vi "2NNN.vi"(11 "Variables and Memory in":T1 {"GFX" format="%02x"}) -> (3 "Variables and Memory out":T1 {"GFX" format="%02x"})   [LabVIEW 2021]
uses:
  Controls/ClusterF.ctl
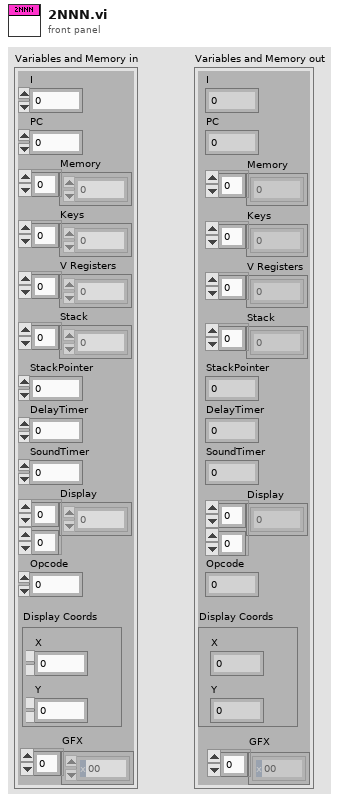
[diagram p1: front panel]
types:
  T1 = typedef "ClusterF.ctl" = cluster{"I":u16, "PC":u16, "Memory":u8[], "Keys":u8[], "V Registers":u8[], "Stack":u16[], "StackPointer":u16, "DelayTimer":u8, "SoundTimer":u8, "Display":u8[][], "Opcode":u16, "Display Coords":cluster{"X":u8, "Y":u8}, "GFX":u8[]}
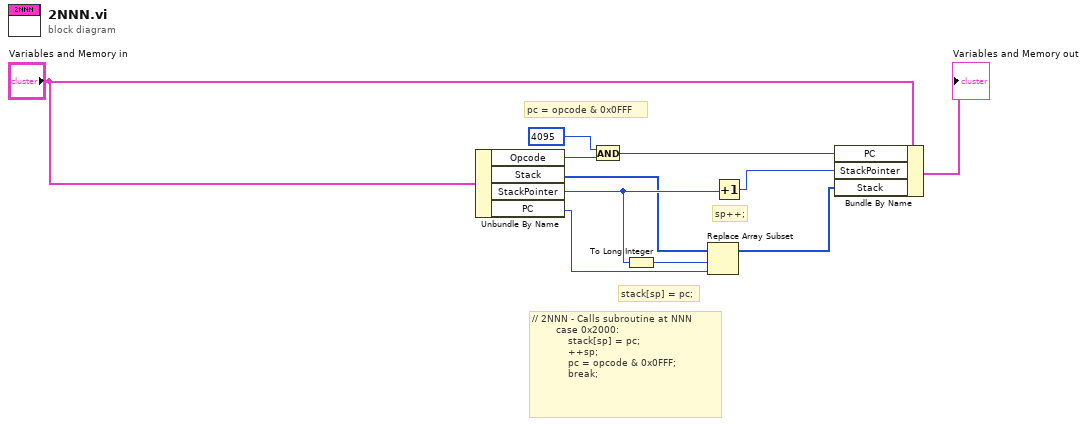
[diagram p0: block diagram]
diagram:
  # "// 2NNN - Calls subroutine at NNN\n        case 0x2000:\n            stack[sp] = pc;\n            ++sp;\n            pc = opcode & 0x0FFF;\n            break;"
  # "pc = opcode & 0x0FFF"
  # "sp++;"
  # "stack[sp] = pc;"
  n1 = Unbundle By Name("Variables and Memory in") -> ("Opcode"=w1:u16, "Stack"=w3:u16[], "StackPointer"=w5:u16, "PC"=w4:u16)
  n2 = And(x=u16 4095 ("y"), y=w1) -> (x .and. y?=w8:u16)
  n3 = To Long Integer(number=w5) -> (32bit integer=w10:i32)
  n4 = Replace Array Subset(array=w3, new element=w4, index=w10) -> (w11:u16[])
  n5 = Increment(x=w5) -> (x+1=w9:u16)
  n6 = Bundle By Name(cluster="Variables and Memory in", "PC"=w8, "StackPointer"=w9, "Stack"=w11) -> (→"Variables and Memory out":T1)
